vi "Deserialize Mission Array.vi"(11 "Serialized Mission Array":string) -> (3 "Mission Object Array":refnum<class "Mission.lvclass">[](array[class]))   [LabVIEW 2011, in "Mission.lvclass"]
uses:
  Mission.lvclass
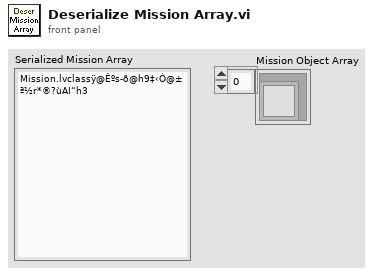
[diagram p1: front panel]
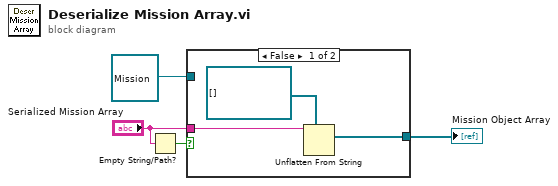
[diagram p0: block diagram]
diagram:
  n1 = Empty String/Path?(string/path="Serialized Mission Array") -> (empty?=w3:bool)
  n2 = case shown="False" w3 {
    tunnel: [w6 _] -> w2
    tunnel: "Serialized Mission Array" -> [w7 _]
    tunnel: refnum<class "Mission.lvclass"> refnum ("Mission.lvclass") -> [_ _]
    frame False {
      n3 = Unflatten From String(type=refnum<class "Mission.lvclass">[] [] ("Mission Object Array"), binary string=w7) -> (value=w6:refnum<class "Mission.lvclass">[])  [unwired: 3 in, 2 out]
    }
    frame True {
    }
  }
  "Mission Object Array" <- w2
